vi "queues1.vi"() -> ()   [LabVIEW 2019]
doc: "This is the first of two demos using Queues. In this demo, one While loop takes the same role as the first loop in the Notifier example, whilst the second While loop plots data. Here, however, the Wait period in the second (consumer) loop is longer than the producer, and so data builds up over time. Because these are using a Queue, the data is not lost - it merely becomes backlogged."
panel:
  out "Consumer":i32
  out "Producer":i32
  in  "stop":bool
  out "Waveform Chart":dbl(graph)
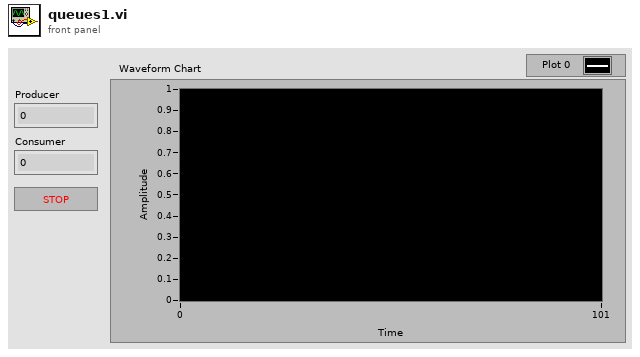
[diagram p1: front panel]
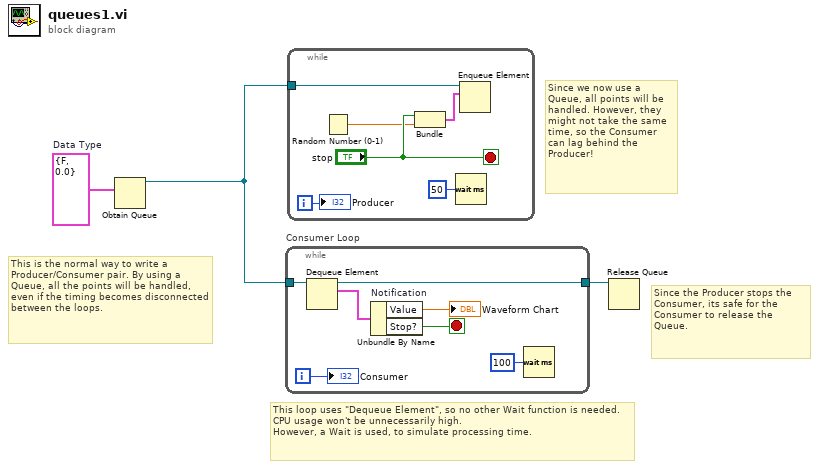
[diagram p0: block diagram]
diagram:
  w3 = cluster{"Stop?":bool, "Value":dbl} {"Stop?"=FALSE, "Value"=0.0}  # Data Type
  # "Since the Producer stops the Consumer, its safe for the Consumer to release the Queue."
  # "This loop uses \"Dequeue Element\", so no other Wait function is needed. CPU usage won't be unnecessarily high.\nHowever, a Wait is used, to simulate processing time."
  # "Since we now use a Queue, all points will be handled. However, they might not take the same time, so the Consumer can lag behind the Producer!"
  # "This is the normal way to write a Producer/Consumer pair. By using a Queue, all the points will be handled, even if the timing becomes disconnected between the loops."
  n1 = Obtain Queue(element data type=w3) -> (queue out=w2:refnum<queue>)  [unwired: 4 in, 2 out]
  n2 = while "Consumer Loop" {
    tunnel: w2 -> [w10]
    tunnel: [w4] -> w1
    i -> [w6]
    stop <- w7 stop-if-true
    n3 = Dequeue Element(queue=w10) -> (queue out=w4:refnum<queue>, element=w9:cluster{"Stop?":bool, "Value":dbl})  [unwired: 2 in, 2 out]
    n4 = Unbundle By Name "Notification"(w9) -> ("Value"=→"Waveform Chart":dbl, "Stop?"=w7:bool)
    n5 = Wait (ms)(milliseconds to wait=u32 100) -> ()  [unwired: 1 out]
    "Consumer" <- w6
  }
  n6 = while {
    tunnel: w2 -> [w16]
    i -> [w11]
    stop <- "stop" stop-if-true
    n7 = Random Number (0-1)() -> (number: 0 to 1=w13:dbl)
    n8 = Bundle("stop"="stop", "number: 0 to 1"=w13) -> (w14:cluster{"stop":bool, "number: 0 to 1":dbl})  [unwired: 1 in]
    n9 = Wait (ms)(milliseconds to wait=u32 50) -> ()  [unwired: 1 out]
    n10 = Enqueue Element(queue=w16, element=w14) -> ()  [unwired: 2 in, 3 out]
    "Producer" <- w11
  }
  n11 = Release Queue(queue=w1) -> ()  [unwired: 2 in, 3 out]
